vi "get channel handle - by device id.vi"(7 "device type":T1=enum."LAN", 8 "error in (no error)":errorcluster, 10 "guid (\"\")":string, 11 "id(0)":u32) -> (0 "error out":errorcluster, 3 "channel handle":u16 format="%x")   [LabVIEW 2024, in "atsj peakcan basic.lvlib"]
doc: "Gets a bus channel handle for a given <b>device type </b>'s device <b>id</b>. Alternatively, if a device <b>guild</b> is provided, it takes precedence over the device id."
uses:
  atsj peakcan basic.lvlib
  device type.ctl
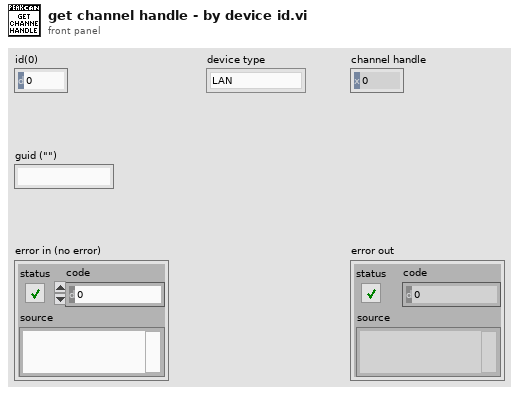
[diagram p1: front panel]
types:
  T1 = typedef "atsj peakcan basic.lvlib/device type.ctl" = enum8{"ISA", "DNG", "PCI", "USB", "PCC", "LAN"}
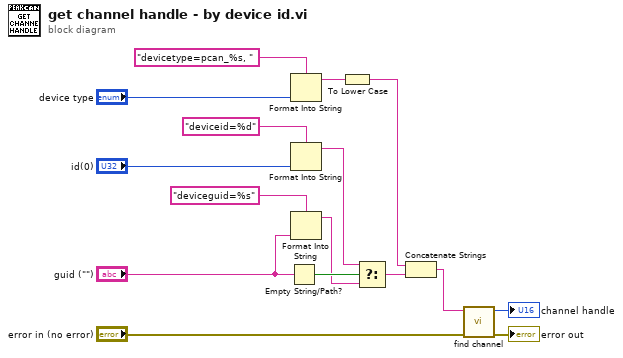
[diagram p0: block diagram]
diagram:
  n1 = Empty String/Path?(string/path="guid (\"\")") -> (empty?=w6:bool)
  n2 = Format Into String(format string="devicetype=pcan_%s, ", "device type") -> (resulting string=w3:string)  [unwired: 2 in, 1 out]
  n3 = Format Into String(format string="deviceid=%d", "id(0)") -> (resulting string=w5:string)  [unwired: 2 in, 1 out]
  n4 = Format Into String(format string="deviceguid=%s", "guid (\"\")") -> (resulting string=w4:string)  [unwired: 2 in, 1 out]
  n5 = To Lower Case(string=w3) -> (all lower case string=w7:string)
  n6 = Select(t=w5, s=w6, f=w4) -> (s? t:f=w2:string)
  n7 = Concatenate Strings(w7, w2) -> (w1:string)
  n8 = call "find channel.vi"("error in (no error)"="error in (no error)", "lookup string"=w1) -> ("error out"=→"error out":errorcluster, "channel handle"=→"channel handle":u16)  [unwired: 8 in]
